vi "Configure Reader.vi"(9 "Packet Msg":refnum<class "Packet Msg.lvclass">, 10 "Rx ID":refnum<k5>, 11 "TCPIP Reader in":refnum<class "TCPIP Reader.lvclass">) -> (3 "TCPIP Reader out":refnum<class "TCPIP Reader.lvclass">)   [LabVIEW 2015, in "TCPIP Reader Actor.lvlib" / "TCPIP Reader.lvclass"]
uses:
  TCPIP Reader.lvclass
  TCPIP Communications Framework/TCPIP Communications Messages/Packet Msg/Packet Msg.lvclass
  TCPIP Reader.lvclass/TCPIP Reader.ctl
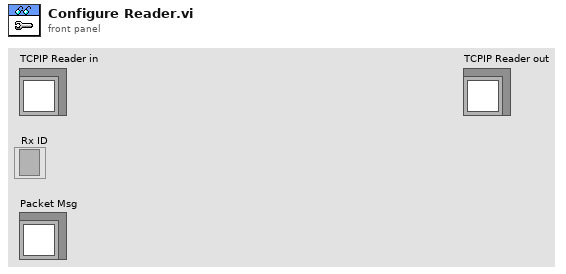
[diagram p1: front panel]
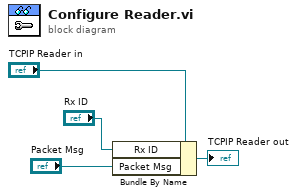
[diagram p0: block diagram]
diagram:
  n1 = Bundle By Name(cluster="TCPIP Reader in", "Rx ID"="Rx ID", "Packet Msg"="Packet Msg") -> (→"TCPIP Reader out":refnum<class "TCPIP Reader.lvclass">)
